vi "JSON Config Single Term Boolean Vector.vi"(7 "Class":refnum<class "Abs_Boolean.lvclass">, 8 "error in (no error)":errorcluster, 11 "Test Value":bool) -> (0 "error out":errorcluster)   [LabVIEW 2021]
uses:
  Source/Abs_Types/Boolean/Abs_Boolean.lvclass
  C:/New folder/LV_Abstract/LV_Abstract/Source/Abs_Types/Type/Abs_Type.lvclass
  Source/Abs_Types/Boolean/Simple Read.vi
  Source/Constants/Support/Bool/Bool.vi
  Source/Functions/Logic/Support/NOT/Bool/Method.vi
  <vilib>/addons/_JKI Toolkits/Caraya/classes/Assert/Assert Equal Value_Variant.vi
  <vilib>/addons/_JKI Toolkits/Caraya/classes/Assert/Assert Equal Type_Variant.vi
  <vilib>/addons/_JKI Toolkits/Caraya/classes/Assert/Assert.lvclass
  <vilib>/addons/_JKI Toolkits/Caraya/classes/Test/Test.lvclass
  <vilib>/Utility/Data Type/NI_Data Type.lvlib
  Source/Abs_Types/Type/Abs_Type.lvclass
  Source/Constants/Support/Bool/Const_Bool.lvclass
  Source/Functions/Logic/Support/NOT/Bool/NOT_Bool.lvclass
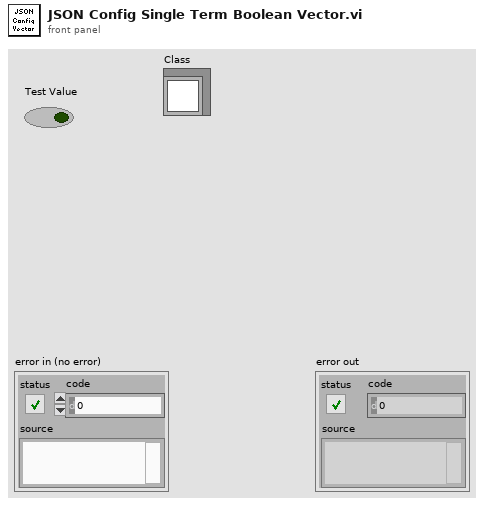
[diagram p1: front panel]
types:
  T1 = typedef "NI_Data Type.lvlib/Data Type.ctl" = enum8{"Invalid Type", "Void", "I8", "I16", "I32", "I64", "U8", "U16", "U32", "U64", "Single Float", "Double Float", "Extended Float", "Single Complex", "Double Complex", "Extended Complex", "Enum U8", "Enum U16", "Enum U32", "Enum U64", "Single Float With Unit", "Double Float With Unit", "Extended Float With Unit", "Single Complex with Unit", "Double Complex with Unit", "Extended Complex with Unit", "Boolean", "String", "Path", "Picture", "Tag", "Array", "Cluster", "Variant", "LV Variant", "Waveform", "Timestamp", "Digital Waveform", "Digital Data", "ExpressData", "Refnum", "External Data", "VI", "Poly VI", "LabVIEW Class Instance", "Fixed Point", "Set Collection", "Map Collection"}
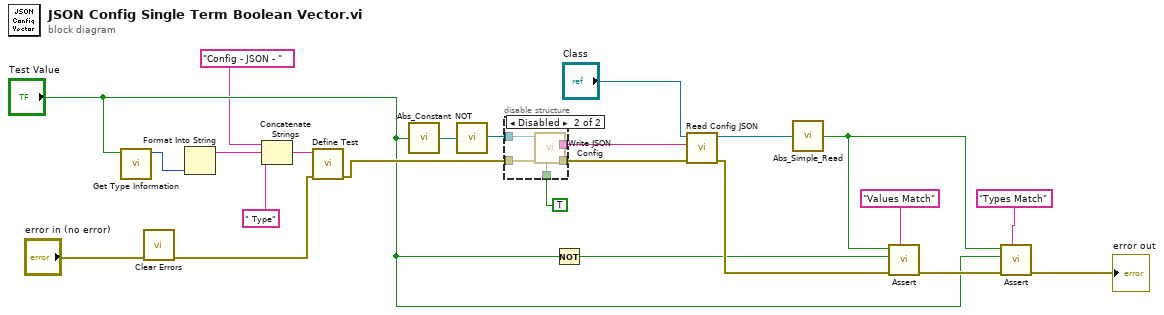
[diagram p0: block diagram]
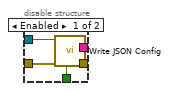
[diagram p2: hidden frame]
diagram:
  n1 = call <vilib>:"Get Type Information.vi"("variant"="Test Value") -> ("type"=w16:T1)  [unwired: 6 in, 4 out]
  n2 = call <vilib>:"Clear Errors.vi"("error in (no error)"="error in (no error)") -> ("error out"=w11:errorcluster)  [unwired: 5 in, 1 out]
  n3 = Format Into String(w16) -> (resulting string=w15:string)  [unwired: 3 in, 1 out]
  n4 = Concatenate Strings("Config - JSON - " ("string"), w15, " Type" ("string")) -> (w14:string)
  n5 = call <vilib>:"Define Test.vi"("error in (no error)"=w11, "Label (VI Title)"=w14) -> ("error out"=w17:errorcluster)  [unwired: 8 in, 1 out]
  n6 = call-poly "Abs_Constant.vi"("Boolean"="Test Value") -> ("Abs_Boolean.lvclass"=w3:refnum<class "Abs_Boolean.lvclass">)  [unwired: 4 in]
  n7 = call-poly "NOT.vi"("Bool"=w3) -> ("Result"=w2:refnum<class "Abs_Boolean.lvclass">)  [unwired: 4 in]
  n8 = disable-structure shown="Disabled" {
    disable-tunnel: w2 -> [w28 w33]
    disable-tunnel: TRUE ("Include Class Name") -> [w27 w32]
    disable-tunnel: [w26 w31] -> w22
    disable-tunnel: [w25 w30] -> w21
    disable-tunnel: w17 -> [w24 w29]
    frame Enabled {
      n9 = call-dynamic "Write JSON Config.vi"("Pretty Print?"=w27, "error in (no error)"=w24, "Abs_Type in"=w28) -> ("error out"=w25:errorcluster, "JSON"=w26:string)  [unwired: 6 in, 1 out]
    }
    frame Disabled {
      n10 = call-dynamic "Write JSON Config.vi"("Pretty Print?"=w32, "error in (no error)"=w29, "Abs_Type in"=w33) -> ("error out"=w30:errorcluster, "JSON"=w31:string)  [unwired: 6 in, 1 out]
    }
  }
  n11 = Not(x="Test Value") -> (.not. x?=w1:bool)
  n12 = call "Read Config JSON.vi"("error in (no error)"=w21, "JSON Config"=w22, "Abs_Type in"="Class") -> ("error out"=w19:errorcluster, "Abs_Type out"=w20:refnum<class "Abs_Boolean.lvclass">)  [unwired: 7 in]
  n13 = call-poly "Abs_Simple_Read.vi"("Boolean in"=w20) -> ("Boolean"=w8:bool)  [unwired: 4 in]
  n14 = call-poly <vilib>:"Assert.vi"("Label"="Values Match", "error in (no error)"=w19, "Actual"=w1, "Expected"=w8) -> ("error out"=w9:errorcluster)  [unwired: 6 in, 1 out]
  n15 = call-poly <vilib>:"Assert.vi"("Label"="Types Match", "error in (no error)"=w9, "Actual"="Test Value", "Expected"=w8) -> ("error out"=→"error out":errorcluster)  [unwired: 6 in, 1 out]
